vi "zc get last error.vi"(8 "error in (no error)":errorcluster, 11 "out":cluster{}) -> (0 "error out":errorcluster, 3 "out out":cluster{})   [LabVIEW 2021, in "zenohc.lvlib"]
doc: "void zc_get_last_error(struct z_view_string_t *out);"
uses:
  zenohc.lvlib
  zenohc.dll
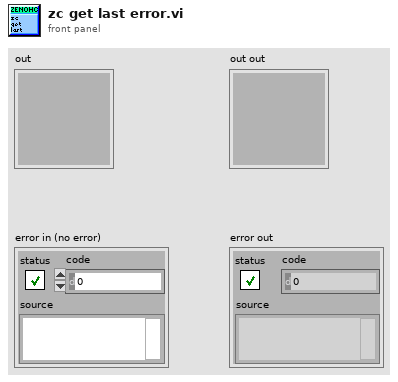
[diagram p1: front panel]
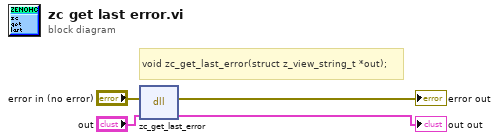
[diagram p0: block diagram]
diagram:
  # "void zc_get_last_error(struct z_view_string_t *out);"
  n1 = dll-call lib="D:/dev/zenoh_labview/zenohc/zenohc.*" fn="zc_get_last_error"(error in="error in (no error)", "out"="out") -> (error out=→"error out":errorcluster, "out"=→"out out":cluster{})  [unwired: 3 in, 1 out]
